vi "NISE.remote.Add Network Chassis.vi"(0 "SLSC Remote in":refnum<class "SLSC Interface.lvclass">, 1 "username":string, 2 "password":string, 5 "chassis IP address/hostname":string, 11 "error in (no error)":errorcluster, 12 "connect timeout (60 sec)":dbl=60.0) -> (4 "SLSC Remote out":refnum<class "SLSC Interface.lvclass">, 6 "chassis out":refnum<k21>, 15 "error out":errorcluster)   [LabVIEW 2016, in "SLSC Interface.lvclass"]
uses:
  SLSC Interface Class/SLSC Interface.lvclass
  SLSC Interface Class/SLSC Interface.lvclass/SLSC Interface.ctl
  SLSC Interface Class/NISE.Read client handle.vi
  SLSC Interface Class/NISE.Read URL.vi
  SLSC Interface Class/NISE.Read session.vi
  <vilib>/httpClient/POSTBuffer.vi
  <vilib>/NI/JSON Support for LabVIEW/JSON Value/Object/Get Value/Get Value (String).vi
  <vilib>/httpClient/LabVIEWHTTPClient.lvlib
  <vilib>/NI/JSON Support for LabVIEW/JSON Value/JSON Value.lvclass
  <vilib>/NI/NI JSONRPC Server Framework/Classes/Client/JSONRPC Client.lvclass
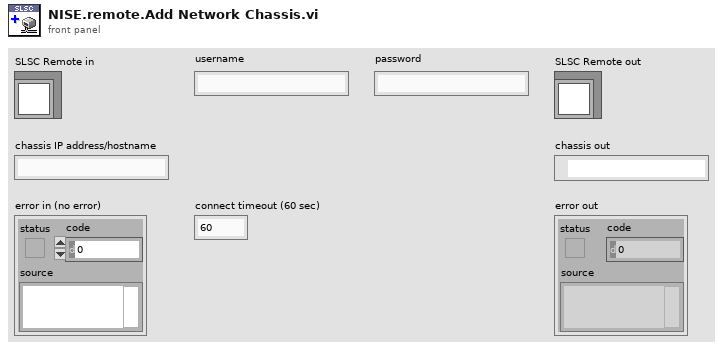
[diagram p1: front panel]
types:
  T1 = typedef "LabVIEWHTTPClient.lvlib/ClientHandle.ctl" = refnum<k1>
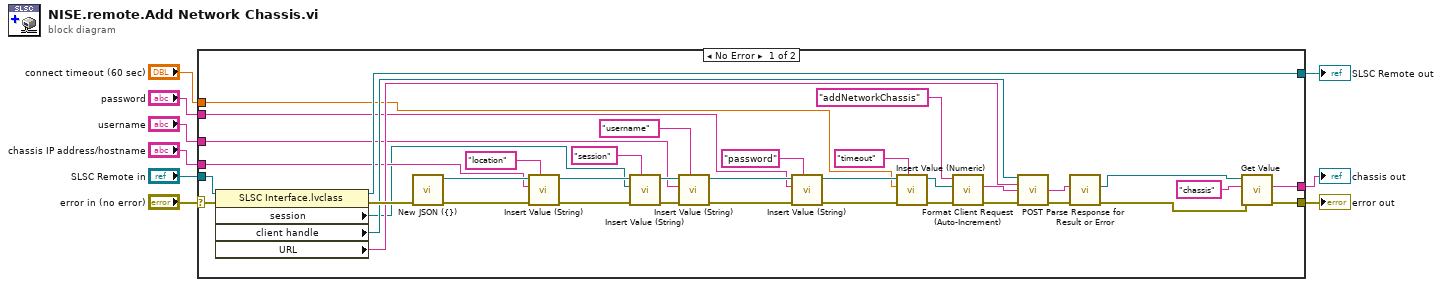
[diagram p0: block diagram]
diagram:
  n1 = case shown="No Error" "error in (no error)" {
    selector: "error in (no error)" -> [w45 w48]
    tunnel: "chassis IP address/hostname" -> [w15 _]
    tunnel: "SLSC Remote in" -> [w47 w49]
    tunnel: [w46 w49] -> w4
    tunnel: [w27 w48] -> w2
    tunnel: "username" -> [w13 _]
    tunnel: "password" -> [w12 _]
    tunnel: "connect timeout (60 sec)" -> [w11 _]
    tunnel: [w28 _] -> w3
    frame No Error {
      n2 = property class="SLSC Interface.lvclass"(reference=w47, error in=w45) -> (reference out=w46:refnum<class "SLSC Interface.lvclass">, error out=w44:errorcluster, "session"=w14:refnum<k21>, "client handle"=w39:T1, "URL"=w38:string)
      n3 = call <vilib>:"New JSON ({}).vi"("error in (no error)"=w44) -> ("error out"=w43:errorcluster, "JSON Value out"=w20:refnum<class "JSON Value.lvclass">)  [unwired: 9 in]
      n4 = call <vilib>:"Insert Value (String).vi"("key"="location" ("Name"), "error in (no error)"=w43, "value"=w15, "JSON Value in"=w20) -> ("error out"=w42:errorcluster, "JSON Value out"=w19:refnum<class "JSON Value.lvclass">)  [unwired: 5 in, 1 out]
      n5 = call <vilib>:"Insert Value (String).vi"("key"="session" ("Name"), "error in (no error)"=w42, "value"=w14, "JSON Value in"=w19) -> ("error out"=w34:errorcluster, "JSON Value out"=w18:refnum<class "JSON Value.lvclass">)  [unwired: 5 in, 1 out]
      n6 = call <vilib>:"Insert Value (String).vi"("key"="username" ("String"), "error in (no error)"=w34, "value"=w13, "JSON Value in"=w18) -> ("error out"=w33:errorcluster, "JSON Value out"=w17:refnum<class "JSON Value.lvclass">)  [unwired: 5 in, 1 out]
      n7 = call <vilib>:"Insert Value (String).vi"("key"="password" ("Name"), "error in (no error)"=w33, "value"=w12, "JSON Value in"=w17) -> ("error out"=w32:errorcluster, "JSON Value out"=w16:refnum<class "JSON Value.lvclass">)  [unwired: 5 in, 1 out]
      n8 = call <vilib>:"Insert Value (Numeric).vi"("key"="timeout" ("Name"), "error in (no error)"=w32, "value"=w11, "JSON Value in"=w16) -> ("error out"=w31:errorcluster, "JSON Value out"=w30:refnum<class "JSON Value.lvclass">)  [unwired: 5 in, 1 out]
      n9 = call <vilib>:"Format Client Request (Auto-Increment).vi"("error in (no error)"=w31, "JSON Value in"=w30, "method"="addNetworkChassis") -> ("error out"=w37:errorcluster, "Request String"=w40:string)  [unwired: 7 in]
      n10 = call-poly <vilib>:"POST.vi"("client handle"=w39, "url"=w38, "buffer"=w40, "error in (no error)"=w37) -> ("body"=w36:string, "error out"=w35:errorcluster)  [unwired: 8 in, 2 out]
      n11 = call <vilib>:"Parse Response for Result or Error.vi"("error in"=w35, "Response String In"=w36) -> ("error out"=w26:errorcluster, "JSON Value out"=w10:refnum<class "JSON Value.lvclass">)  [unwired: 7 in, 1 out]
      n12 = call-poly <vilib>:"Get Value.vi"("error in (no error)"=w26, "key"="chassis" ("Parameter Name"), "JSON Value in"=w10) -> ("error out"=w27:errorcluster, "value"=w28:string)  [unwired: 7 in]
    }
    frame Error {
    }
  }
  "error out" <- w2
  "SLSC Remote out" <- w4
  "chassis out" <- w3
